vi "MC5e Check Squad Name Unique.vi"(6 "index":i32, 7 "Mode":T1, 8 "error in":errorcluster, 11 "Squad Name":string) -> (0 "error out":errorcluster, 2 "Squad Name is Unique and non-blank":bool, 3 "OK Button Disabled?":T2(ring))   [LabVIEW 2020]
uses:
  MC5e Editor modes.ctl
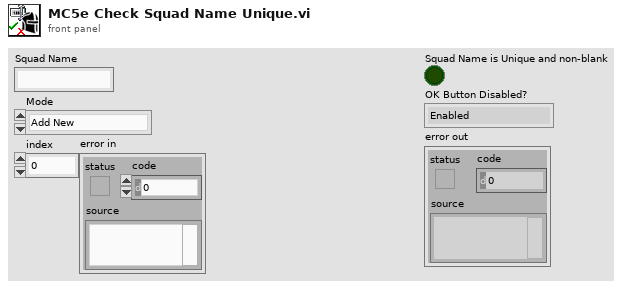
[diagram p1: front panel]
types:
  T1 = typedef "MC5e Editor modes.ctl" = enum16{"Add New", "Copy Selected", "Delete Selected", "Edit Selected"}
  T2 = enum8{"Enabled", "Disabled", "Disabled and Grayed Out"}
  T3 = typedef "MC5e Squad_Info.ctl" = cluster{"Squad Name":string, "# Soldiers":u16, "Battle Rating":u16, "Flying":bool, "Mounted":bool, "Speed":u16, "Range":u16, "Morale":i32, "Max Endurance":u16, "Current Endurance":i32, "Size":T4, "Space Taken":u16, "Difficult Terrain":i32[], "CR":u16, "Special / Notes":string}
  T4 = typedef "MC5e Size_Categories.ctl" = enum16{"Tiny", "Small", "Medium", "Large", "Huge", "Gargantuan"}
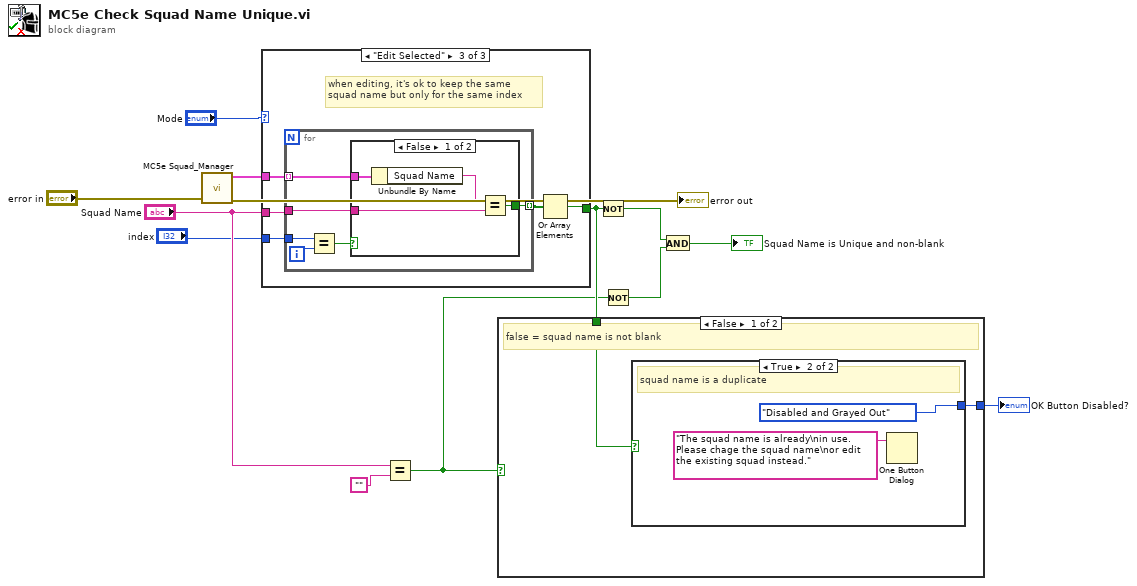
[diagram p0: block diagram]
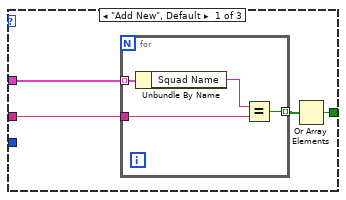
[diagram p2: hidden frame]
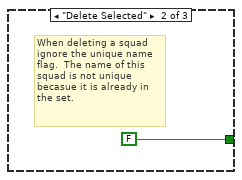
[diagram p3: hidden frame]
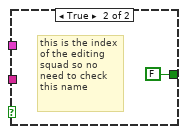
[diagram p4: hidden frame]
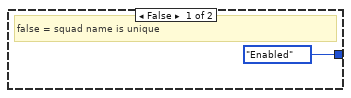
[diagram p5: hidden frame]
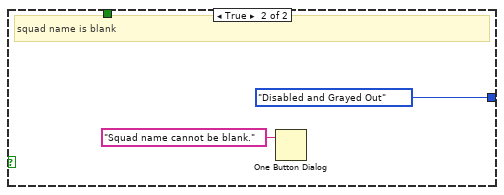
[diagram p6: hidden frame]
diagram:
  n1 = call "MC5e Squad_Manager.vi"("error in"="error in") -> ("error out"=→"error out":errorcluster, "All Squads Out"=w3:T3[])  [unwired: 7 in, 2 out]
  n2 = case shown="\"Edit Selected\"" "Mode" {
    tunnel: w3 -> [w17 _ w26]
    tunnel: [w15 FALSE w24] -> w12
    tunnel: "Squad Name" -> [w14 _ w25]
    tunnel: "index" -> [_ _ w23]
    frame "Add New", Default {
      n3 = for {
        tunnel: w17 -> [w21] mode=indexing
        tunnel: [w19] -> w16 mode=indexing
        tunnel: w14 -> [w18]
        n4 = Unbundle By Name(w21) -> ("Squad Name"=w20:string)
        n5 = Equal?(x=w20, y=w18) -> (x = y?=w19:bool)
      }
      n6 = Or Array Elements(Boolean array=w16) -> (logical OR=w15:bool)
    }
    frame "Delete Selected" {
      # "When deleting a squad\nignore the unique name\nflag.  The name of this\nsquad is not unique \nbecasue it is already in\nthe set."
    }
    frame "Edit Selected" {
      # "when editing, it's ok to keep the same\nsquad name but only for the same index"
      n7 = for {
        tunnel: w26 -> [w33] mode=indexing
        tunnel: [w32] -> w27 mode=indexing
        tunnel: w25 -> [w31]
        tunnel: w23 -> [w29]
        i -> [w30]
        n8 = Equal?(x=w29, y=w30) -> (x = y?=w28:bool)
        n9 = case shown="False" w28 {
          tunnel: w33 -> [w37 _]
          tunnel: [w35 FALSE] -> w32
          tunnel: w31 -> [w34 _]
          frame False {
            n10 = Unbundle By Name(w37) -> ("Squad Name"=w36:string)
            n11 = Equal?(x=w36, y=w34) -> (x = y?=w35:bool)
          }
          frame True {
            # "this is the index\nof the editing\nsquad so no \nneed to check\nthis name"
          }
        }
      }
      n12 = Or Array Elements(Boolean array=w27) -> (logical OR=w24:bool)
    }
  }
  n13 = Equal?(x="Squad Name", y="") -> (x = y?=w8:bool)
  n14 = case shown="False" w8 {
    tunnel: w12 -> [w40 _]
    tunnel: [w39 T2."Disabled and Grayed Out" ("Disabled")] -> w11
    frame False {
      # "false = squad name is not blank"
      n15 = case shown="True" w40 {
        tunnel: [T2."Enabled" ("Disabled") T2."Disabled and Grayed Out" ("Disabled")] -> w39
        frame False {
          # "false = squad name is unique"
        }
        frame True {
          # "squad name is a duplicate"
          n16 = One Button Dialog(message="The squad name is already\nin use.  Please chage the squad name\nor edit the existing squad instead.") -> ()  [unwired: 1 in, 1 out]
        }
      }
    }
    frame True {
      # "squad name is blank"
      n17 = One Button Dialog(message="Squad name cannot be blank.") -> ()  [unwired: 1 in, 1 out]
    }
  }
  "OK Button Disabled?" <- w11
  n18 = Not(x=w12) -> (.not. x?=w13:bool)
  n19 = Not(x=w8) -> (.not. x?=w6:bool)
  n20 = And(x=w13, y=w6) -> (x .and. y?=→"Squad Name is Unique and non-blank":bool)
